vi "RTS Get Section List.vi"(8 "Error In":errorcluster, 10 "Section Name":string, 11 "Sorted Array":string[](array[string])) -> (0 "Error Out":errorcluster, 3 "Parsed Array":string[](array[string]))   [LabVIEW 2016]
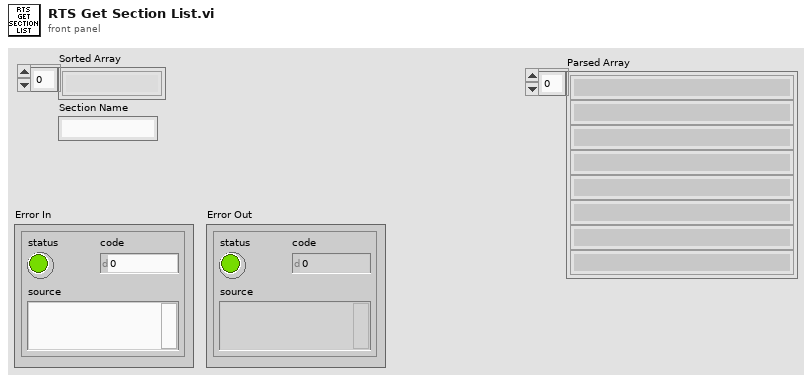
[diagram p1: front panel]
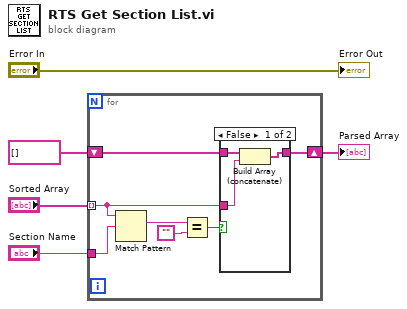
[diagram p0: block diagram]
diagram:
  n1 = for {
    tunnel: "Sorted Array" -> [w7] mode=indexing
    shift-right: [w8] -> w3
    shift-left: string[] [] -> [w9]
    tunnel: "Section Name" -> [w6]
    n2 = Match Pattern(string=w7, regular expression=w6) -> (match substring=w12:string)  [unwired: 1 in, 3 out]
    n3 = Equal?(x=w12, y="") -> (x = y?=w10:bool)
    n4 = case shown="False" w10 {
      tunnel: w9 -> [w15 w16]
      tunnel: [w13 w16] -> w8
      tunnel: w7 -> [w14 _]
      frame False {
        n5 = Build Array (concatenate)(w15, w14) -> (w13:string[])
      }
      frame True {
      }
    }
  }
  "Parsed Array" <- w3
  "Error Out" <- "Error In"
